vi "TENT O2 SENSOR.vi"() -> ()   [LabVIEW 2016]
uses:
  <vilib>/DAQmx/read.llb/DAQmx Read (Analog DBL 1Chan 1Samp).vi
  <vilib>/DAQmx/miscellaneous.llb/DAQmx Fill In Error Info.vi
panel:
  out "Current PPM":dbl
  out "Voltage Out":dbl
  out "This is good data!!":bool
  out "O2 PPM":dbl(graph)
  in  "stop":bool
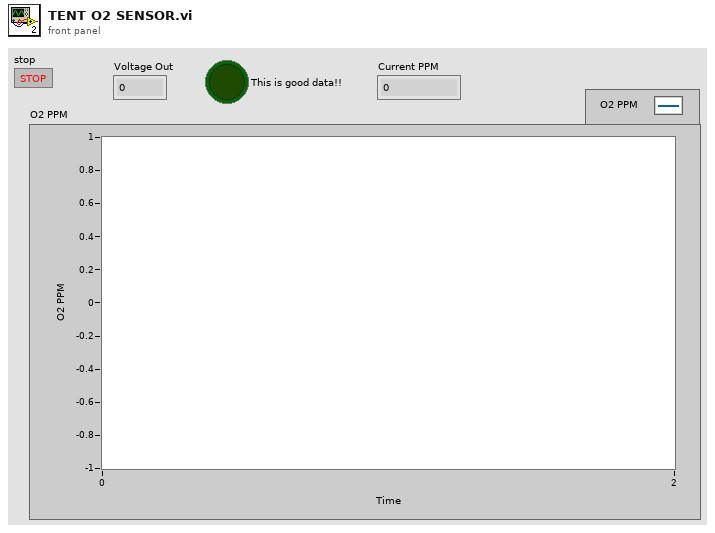
[diagram p1: front panel]
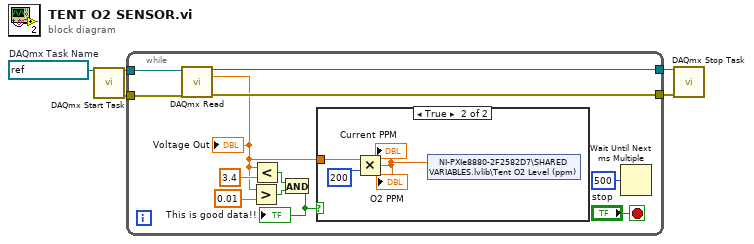
[diagram p0: block diagram]
diagram:
  w4 = refnum<k21> "o2voltage"  # DAQmx Task Name
  n1 = call <vilib>:"DAQmx Start Task.vi"("task/channels in"=w4) -> ("task out"=w3:refnum<k21>, "error out"=w5:errorcluster)  [unwired: 13 in]
  n2 = while {
    tunnel: [w17] -> w1
    tunnel: [w15] -> w2
    tunnel: w3 -> [w9]
    tunnel: w5 -> [w8]
    stop <- "stop" stop-if-true
    n3 = call-poly <vilib>:"DAQmx Read.vi"("task/channels in"=w9, "error in"=w8) -> ("task out"=w17:refnum<k21>, "data"=w6:dbl, "error out"=w15:errorcluster)  [unwired: 11 in]
    "Voltage Out" <- w6
    n4 = Greater?(x=w6, y=0.01) -> (0:w11:bool)
    n5 = Less?(x=w6, y=3.4) -> (x < y?=w13:bool)
    n6 = And(x=w13, y=w11) -> (x .and. y?=w10:bool)
    "This is good data!!" <- w10
    n7 = case shown="True" w10 {
      tunnel: w6 -> [_ w20]
      frame False {
      }
      frame True {
        n8 = Multiply(x=w20, y=200) -> (x*y=w18:dbl)
        "O2 PPM" <- w18
        "Current PPM" <- w18
        n9 = shared-variable "NI-PXIe8880-2F2582D7\\SHARED VARIABLES.lvlib\\Tent O2 Level (ppm)"(w18) -> ()  [unwired: 1 in, 1 out]
      }
    }
    n10 = Wait Until Next ms Multiple(millisecond multiple=u32 500) -> ()  [unwired: 1 out]
  }
  n11 = call <vilib>:"DAQmx Stop Task.vi"("task/channels in"=w1, "error in"=w2) -> ()  [unwired: 12 in, 2 out]
